vi "Configure RTD [RTD].vi"(8 "error in (no error)":errorcluster, 9 "resistance (0.0 ohms)":dbl format="%^.2e", 10 "alpha (0.0)":dbl format="%^.2e", 11 "IVI_DMM in":refnum<class "IVI_DMM.lvclass">) -> (0 "error out":errorcluster, 3 "IVI_DMM out":refnum<class "IVI_DMM.lvclass">)   [LabVIEW 2013, in "IVI_DMM.lvlib" / "IVI_DMM.lvclass"]
doc: "This VI configures the alpha and resistance parameters for a resistance temperature device.\n\nThis VI affects the behavior of the instrument only when the IviDmm>Temperature Measurements>Transducer Type [TMP] property is set to IVIDMM_VAL_2_WIRE_RTD or IVIDMM_VAL_4_WIRE_RTD.\n\nNote:\n\n(1) This VI is part of the IviDmmResistanceTemperatureDevice [RTD] extension group.\n\n(2) The driver assumes that you are using a Platinum Resistance Temperature Device."
uses:
  IVI_DMM.lvclass
  IVI_DMM.lvclass/IVI_DMM.ctl
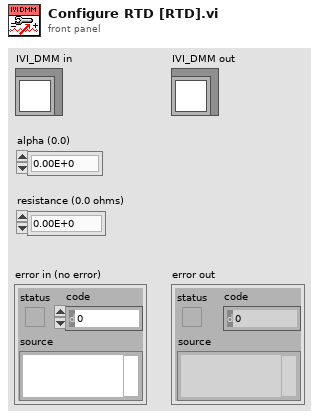
[diagram p1: front panel]
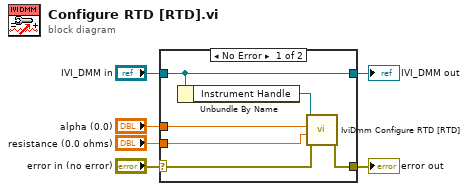
[diagram p0: block diagram]
diagram:
  n1 = case shown="No Error" "error in (no error)" {
    selector: "error in (no error)" -> [w9 w14]
    tunnel: [w11 w14] -> w5
    tunnel: [w12 w13] -> w3
    tunnel: "IVI_DMM in" -> [w12 w13]
    tunnel: "alpha (0.0)" -> [w8 _]
    tunnel: "resistance (0.0 ohms)" -> [w7 _]
    frame No Error {
      n2 = Unbundle By Name(w12) -> ("Instrument Handle"=w10:refnum<k15>)
      n3 = call <vilib>:"IviDmm Configure RTD [RTD].vi"("error in (no error)"=w9, "resistance (0.0 ohms)"=w7, "alpha (0.0)"=w8, "instrument handle"=w10) -> ("error out"=w11:errorcluster)  [unwired: 6 in, 1 out]
    }
    frame Error {
    }
  }
  "error out" <- w5
  "IVI_DMM out" <- w3
